vi "test 04 - ARInit.vi"() -> ()   [LabVIEW 2020]
uses:
  UI_Actor/UI_Actor/ctl_AR_Parameters.ctl
  UI_Actor/UI_Actor/ctl_AR_Mode.ctl
  support/Databox.lvlibp/TypesTools/Config/Config.lvclass
  support/Databox.lvlibp/TypesTools/Data/Data.lvclass
  support/Databox.lvlibp/TypesTools/Data/TypeEnum.ctl
  UIA_UTsupport/UIA_UTsupport.lvclass
  D:/Projets/STEP AT/UI Actor/UI_Actor/UI_Actor/UI_Actor.lvclass
  UI_Actor/UI_Actor Messages/UI_AutoRefresh Msg/UI_AutoRefresh Msg.lvclass/UI_AutoRefresh Msg.ctl
  f7e9fdf2-272c-4cde-b3ea-907668245b3f.vi
  e3e33372-f0f8-45c8-a109-52282a8919ad.vi
  4179e056-1b7e-4481-8e47-4e54562ce6c4.vi
  UIA_UTsupport/gloglo.vi
  support/Actor Framework.lvlibp/1abvi3w/vi.lib/ActorFramework/Message Enqueuer/Enqueue.vi
  UI_Actor/UI_Actor Messages/UI_AutoRefresh Msg/UI_AutoRefresh Msg.lvclass
  UI_Actor/UI_Actor/UI_Actor.lvclass
  support/Actor Framework.lvlibp/1abvi3w/vi.lib/ActorFramework/Stop Msg/Stop Msg.lvclass
panel:
  out "PASS":bool
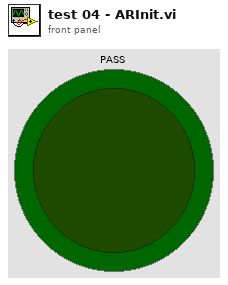
[diagram p1: front panel]
types:
  T1 = typedef "Databox.lvlibp/Data.lvclass/TypeEnum.ctl" = enum16{"Boolean", "SByte", "Byte", "Int16", "UInt16", "Int32", "UInt32", "Int64", "UInt64", "Float", "Double", "String", "DateTime", "ByteString", "Array of Boolean", "Array of SByte", "Array of Byte", "Array of Int16", "Array of UInt16", "Array of Int32", "Array of UInt32", "Array of Int64", "Array of UInt64", "Array of Float", "Array of Double", "Array of String", "Array of DateTime", "Array of ByteString", "Matrix of Boolean", "Matrix of SByte", "Matrix of Byte", "Matrix of Int16", "Matrix of UInt16", "Matrix of Int32", "Matrix of UInt32", "Matrix of Int64", "Matrix of UInt64", "Matrix of Float", "Matrix of Double", "Matrix of String ", "Matrix of DateTime", "Matrix of ByteString"}
  T2 = cluster{"Ch.Conf":refnum<class "Config.lvclass">, "Data":refnum<class "Data.lvclass">[]}
  T3 = typedef "UI_Actor.lvlib/UI_Actor.lvclass/ctl_AR_Parameters.ctl" = cluster{"Write TipStrips with details (T)":bool, "Write Captions with UserLabels (T)":bool, "Mode (ind only)":T4, "Enable nested stream (T)":bool}
  T4 = typedef "UI_Actor.lvlib/UI_Actor.lvclass/ctl_AR_Mode.ctl" = enum16{"Controls only", "Indicators only", "All"}
  T5 = cluster{"Ch.Conf":refnum<class "Config.lvclass">, "Data":refnum<class "Data.lvclass">[]}[]
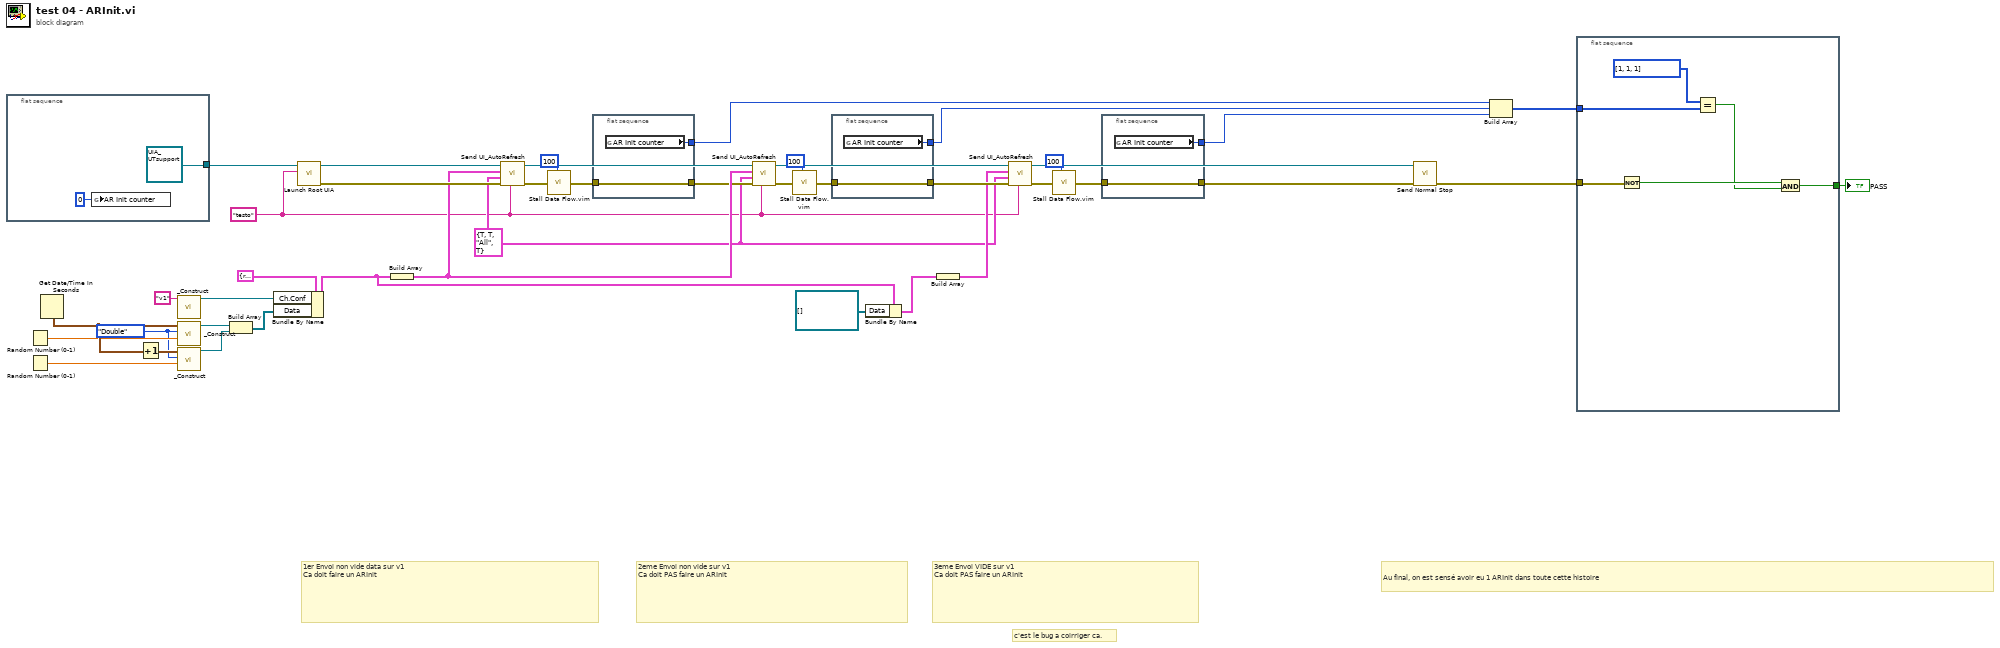
[diagram p0: block diagram]
diagram:
  w27 = TypeEnum."Double" ("Type")
  w8 = "testo" ("Actor Name")
  w9 = T3 {"Write TipStrips with details (T)"=TRUE, "Write Captions with UserLabels (T)"=TRUE, "Mode (ind only)"=enum."All", "Enable nested stream (T)"=TRUE} ("Parameters (Tipstrips,Captions,All)")
  # "c'est le bug a coirriger ca."
  # "3eme Envoi VIDE sur v1\nCa doit PAS faire un ARInit"
  # "2eme Envoi non vide sur v1\nCa doit PAS faire un ARInit"
  # "Au final, on est sensé avoir eu 1 ARInit dans toute cette histoire"
  # "1er Envoi non vide data sur v1\nCa doit faire un ARInit"
  n1 = flat-sequence {
    tunnel: [refnum<class "UIA_UTsupport.lvclass"> refnum ("UIA_UTsupport.lvlib:UIA_UTsupport.lvclass")] -> w26
    frame #0 {
      n2 = global write "gloglo.vi" "AR Init counter"(0 ("AR Init counter")) -> ()
    }
  }
  n3 = Random Number (0-1)() -> (number: 0 to 1=w30:dbl)
  n4 = Random Number (0-1)() -> (number: 0 to 1=w28:dbl)
  n5 = Get Date/Time In Seconds() -> (seconds since 1Jan1904=w32:timestamp)
  n6 = Increment(x=w32) -> (x+1=w31:timestamp)
  n7 = call "_Construct.vi"("System Label"="v1") -> ("Ch.Conf out"=w41:refnum<class "Config.lvclass">)  [unwired: 13 in, 1 out]
  n8 = call "_Construct.vi"("Value"=w30, "Type"=w27, "Time (now!)"=w32) -> ("Ch.TData out"=w40:refnum<class "Data.lvclass">)  [unwired: 7 in, 1 out]
  n9 = call "_Construct.vi"("Value"=w28, "Type"=w27, "Time (now!)"=w31) -> ("Ch.TData out"=w39:refnum<class "Data.lvclass">)  [unwired: 7 in, 1 out]
  n10 = Build Array(w40, w39) -> (w38:refnum<class "Data.lvclass">[])
  n11 = Bundle By Name(cluster=T2 {"Ch.Conf"=refnum, "Data"=[]} ("Cluster"), "Ch.Conf"=w41, "Data"=w38) -> (w13:T2)
  n12 = call "Launch Root UIA.vi"("Actor Name"=w8, "UI_Actor in"=w26) -> ("error out"=w42:errorcluster, "Actor's Enqueuer"=w36:refnum<class "Message Enqueuer.lvclass">)  [unwired: 8 in]
  n13 = Build Array(w13) -> (w25:T5)
  n14 = call "Send UI_AutoRefresh.vi"("Sourcer name"=w8, "error in (no error)"=w42, "Parameters (Tipstrips,Captions,All)"=w9, "Data chunk"=w25, "Message Enqueuer"=w36) -> ("error out"=w24:errorcluster, "Message Enqueuer out"=w33:refnum<class "Message Enqueuer.lvclass">)  [unwired: 5 in]
  n15 = call "Stall Data Flow.vim"("value in"=w24, "milliseconds to wait"=u32 100) -> ("value out"=w21:errorcluster)  [unwired: 1 out]
  n16 = flat-sequence {
    tunnel: [w46] -> w22
    tunnel: w21 -> [w46]
    tunnel: [w45] -> w20
    frame #0 {
      n17 = global read "gloglo.vi" "AR Init counter"() -> (w45:i32)
    }
  }
  n18 = call "Send UI_AutoRefresh.vi"("Sourcer name"=w8, "error in (no error)"=w22, "Parameters (Tipstrips,Captions,All)"=w9, "Data chunk"=w25, "Message Enqueuer"=w33) -> ("error out"=w2:errorcluster, "Message Enqueuer out"=w17:refnum<class "Message Enqueuer.lvclass">)  [unwired: 5 in]
  n19 = call "Stall Data Flow.vim"("value in"=w2, "milliseconds to wait"=u32 100) -> ("value out"=w1:errorcluster)  [unwired: 1 out]
  n20 = flat-sequence {
    tunnel: [w48] -> w16
    tunnel: w1 -> [w48]
    tunnel: [w47] -> w19
    frame #0 {
      n21 = global read "gloglo.vi" "AR Init counter"() -> (w47:i32)
    }
  }
  n22 = Bundle By Name(cluster=w13, "Data"=refnum<class "Data.lvclass">[] []) -> (w11:T2)
  n23 = Build Array(w11) -> (w10:T5)
  n24 = call "Send UI_AutoRefresh.vi"("Sourcer name"=w8, "error in (no error)"=w16, "Parameters (Tipstrips,Captions,All)"=w9, "Data chunk"=w10, "Message Enqueuer"=w17) -> ("error out"=w4:errorcluster, "Message Enqueuer out"=w15:refnum<class "Message Enqueuer.lvclass">)  [unwired: 5 in]
  n25 = call "Stall Data Flow.vim"("value in"=w4, "milliseconds to wait"=u32 100) -> ("value out"=w3:errorcluster)  [unwired: 1 out]
  n26 = flat-sequence {
    tunnel: [w50] -> w14
    tunnel: w3 -> [w50]
    tunnel: [w49] -> w7
    frame #0 {
      n27 = global read "gloglo.vi" "AR Init counter"() -> (w49:i32)
    }
  }
  n28 = call "Send Normal Stop.vi"("error in (no error)"=w14, "Message Enqueuer"=w15) -> ("error out"=w34:errorcluster)  [unwired: 9 in]
  n29 = Build Array(w20, w19, w7) -> (w18:i32[])
  n30 = flat-sequence {
    tunnel: w34 -> [w56]
    tunnel: [w54] -> w35
    tunnel: w18 -> [w53]
    frame #0 {
      n31 = Not(x=w56) -> (.not. x?=w55:bool)
      n32 = Equal?(x=i32[] [1, 1, 1], y=w53) -> (x = y?=w52:bool)
      n33 = And(x=w55, y=w52) -> (x .and. y?=w54:bool)
    }
  }
  "PASS" <- w35
